vi "CreateFakeTestListener.vi"(8 "error in (no error)":errorcluster) -> (0 "error out":errorcluster, 3 "FakeTestListener":refnum<class "FakeTestListener.lvclass">)   [LabVIEW 2017, in "TestResult.Tests.lvlib" / "Support.lvlib" / "FakeTestListener.lvclass"]
uses:
  FakeTestListener.lvclass
  FakeTestListener.lvclass/FakeTestListener.ctl
panel:
  in  "FakeTestListener In":refnum<class "FakeTestListener.lvclass">
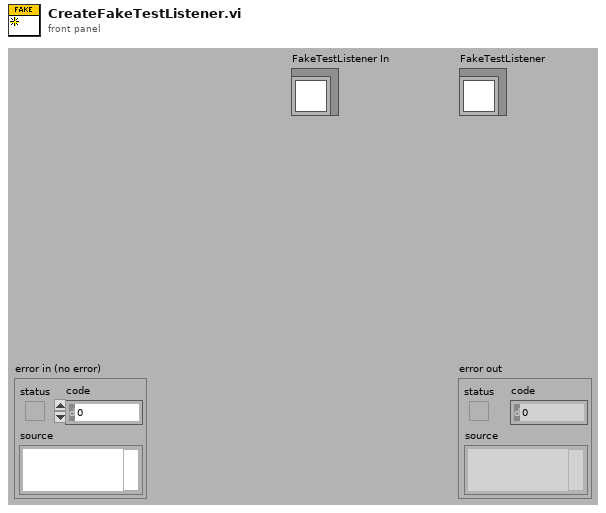
[diagram p1: front panel]
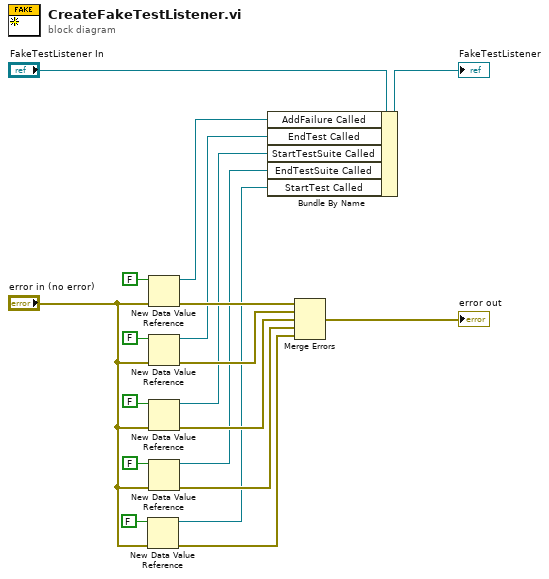
[diagram p0: block diagram]
diagram:
  n1 = New Data Value Reference(data value=FALSE, error in="error in (no error)") -> (data value reference=w1:refnum<data-value>, error out=w2:errorcluster)
  n2 = New Data Value Reference(data value=FALSE, error in="error in (no error)") -> (data value reference=w17:refnum<data-value>, error out=w13:errorcluster)
  n3 = New Data Value Reference(data value=FALSE, error in="error in (no error)") -> (data value reference=w12:refnum<data-value>, error out=w14:errorcluster)
  n4 = New Data Value Reference(data value=FALSE, error in="error in (no error)") -> (data value reference=w8:refnum<data-value>, error out=w9:errorcluster)
  n5 = New Data Value Reference(data value=FALSE, error in="error in (no error)") -> (data value reference=w5:refnum<data-value>, error out=w6:errorcluster)
  n6 = Bundle By Name(cluster="FakeTestListener In", "AddFailure Called"=w17, "EndTest Called"=w12, "StartTestSuite Called"=w8, "EndTestSuite Called"=w5, "StartTest Called"=w1) -> (→"FakeTestListener":refnum<class "FakeTestListener.lvclass">)
  n7 = Merge Errors(w13, w14, w9, w6, w2) -> (→"error out":errorcluster)
